vi "Wrap.vi"(7 "Actor in":refnum<class "Actor.lvclass">, 8 "Error in":errorcluster, 10 "Msg DVR in":refnum<data-value>, 11 "TEMPLATE Msg in":refnum<class "TEMPLATE Msg.lvclass">) -> (0 "Error out":errorcluster, 2 "Msg DVR out":refnum<data-value>, 5 "Actor out":refnum<class "Actor.lvclass">)   [LabVIEW 2020, in "_Template.lvlib" / "Templates.lvlib" / "TEMPLATE jettl Msg.lvlib" / "TEMPLATE Msg.lvclass"]
uses:
  TEMPLATE Msg.lvclass
  TEMPLATE Msg.lvclass/TEMPLATE Msg.ctl
  jettl/jettl/Msg/Msg.lvclass
  jettl/jettl/Msg Contents/Msg Contents.lvclass
  jettl/jettl/Msg Output/Msg Output.lvclass
  TEMPLATE Msg Contents/TEMPLATE Msg Contents.lvclass
  jettl/jettl/Actor/Actor.lvclass
  jettl/jettl/Msg.ctl
  jettl/jettl/jettl.lvlib
  jettl/jettl/Teller.ctl
  jettl/jettl/Unified Actor Relation.ctl
panel:
  # "This front panel should not be manipulated."
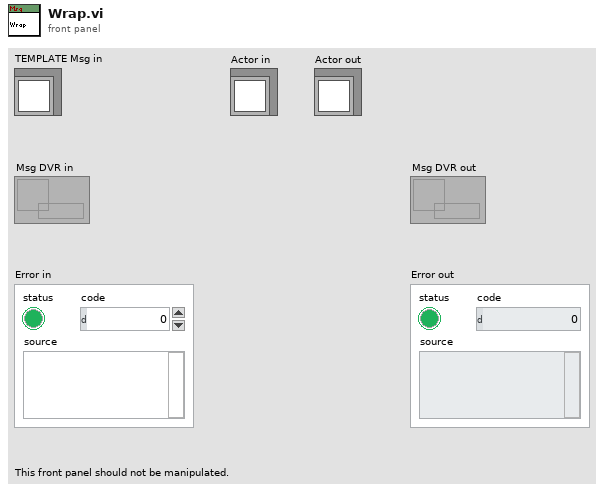
[diagram p1: front panel]
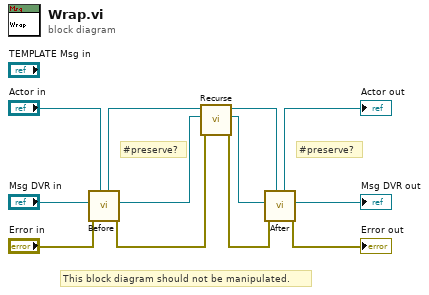
[diagram p0: block diagram]
diagram:
  # "#preserve?"
  # "#preserve?"
  # "This block diagram should not be manipulated."
  n1 = call "Before.vi"("Actor in"="Actor in", "Error in"="Error in", "Msg DVR in"="Msg DVR in") -> ("Error out"=w6:errorcluster, "Msg DVR out"=w3:refnum<data-value>, "Actor out"=w8:refnum<class "Actor.lvclass">)  [unwired: 6 in]
  n2 = call-dynamic "Recurse.vi"("Error in"=w6, "Msg DVR in"=w3, "Actor in"=w8) -> ("Error out"=w5:errorcluster, "Msg DVR out"=w2:refnum<data-value>, "Actor out"=w7:refnum<class "Actor.lvclass">)  [unwired: 6 in]
  n3 = call "After.vi"("Actor in"=w7, "Error in"=w5, "Msg DVR in"=w2) -> ("Error out"=→"Error out":errorcluster, "Msg DVR out"=→"Msg DVR out":refnum<data-value>, "Actor out"=→"Actor out":refnum<class "Actor.lvclass">)  [unwired: 6 in]
